vi "Temperature.vi"(0 "physical channels":tag="PXI1Slot2/ai2", 1 "current excitation value":dbl=0.0009 format="%0.5f", 2 "r0":dbl=100.0 format="%0.2f", 5 "current excitation source":i32(ring)=10200 items=["Internal"=10200, "External"=10167, "None"=10230], 7 "resistance configuration":i32(ring)=2 items=["2-Wire"=2, "3-Wire"=3, "4-Wire"=4], 9 "rtd type":i32(ring)=10071 items=["Pt3750"=12481, "Pt3851"=10071, "Pt3911"=12482, "Pt3916"=10069, "Pt3920"=10053, "Pt3928"=12483, "Custom"=10137], 11 "units":i32(ring)=10143 items=["Deg C"=10143, "Deg F"=10144, "Kelvins"=10325, "Deg R"=10145, "From Custom Scale"=10065], 12 "minimum value":dbl format="%0.2f", 13 "maximum value":dbl=100.0 format="%0.2f") -> (4 "data":dbl[](array[numeric]) format="%0.2f", 15 "error out":errorcluster)   [LabVIEW 2019]
uses:
  <vilib>/DAQmx/read.llb/DAQmx Read (Analog 1D DBL NChan 1Samp).vi
  <vilib>/DAQmx/create/channels.llb/DAQmx Create Channel (AI-Temperature-RTD).vi
  <vilib>/DAQmx/miscellaneous.llb/DAQmx Fill In Error Info.vi
panel:
  out "Waveform Chart":dbl[](graph)
  # "Para el NI PXIe-4357"
  # "chanel 2 (ai2) for rtd"
  # "Pt3851 for rtd"
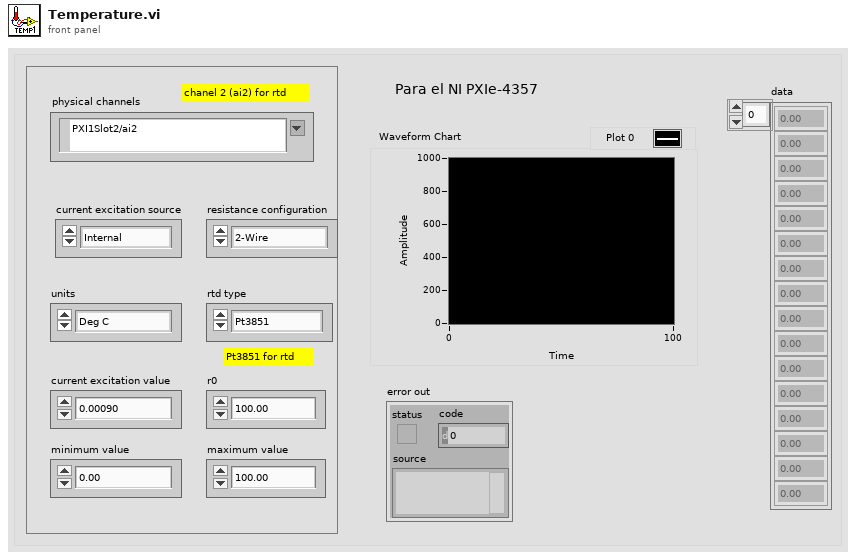
[diagram p1: front panel]
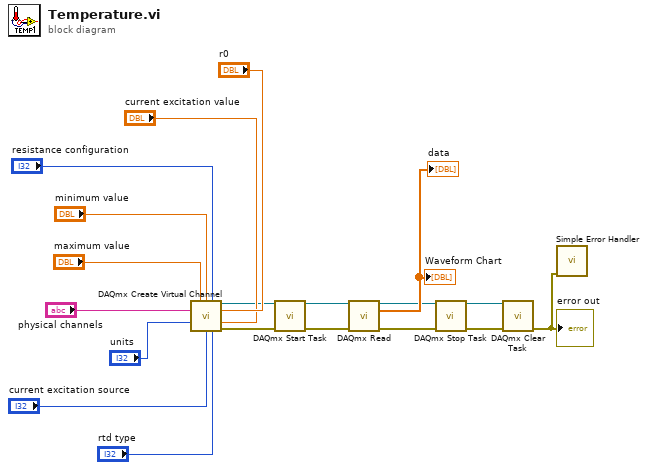
[diagram p0: block diagram]
diagram:
  n1 = call-poly <vilib>:"DAQmx Create Virtual Channel.vi"("maximum value"="maximum value", "minimum value"="minimum value", "resistance configuration"="resistance configuration", "physical channels"="physical channels", "r0"="r0", "units"="units", "current excitation value"="current excitation value", "current excitation source"="current excitation source", "rtd type"="rtd type") -> ("task out"=w3:refnum<k21>, "error out"=w4:errorcluster)  [unwired: 5 in]
  n2 = call <vilib>:"DAQmx Start Task.vi"("task/channels in"=w3, "error in"=w4) -> ("task out"=w5:refnum<k21>, "error out"=w6:errorcluster)  [unwired: 12 in]
  n3 = call-poly <vilib>:"DAQmx Read.vi"("task/channels in"=w5, "error in"=w6) -> ("task out"=w7:refnum<k21>, "data"=→"Waveform Chart" →"data":dbl[], "error out"=w8:errorcluster)  [unwired: 11 in]
  n4 = call <vilib>:"DAQmx Stop Task.vi"("task/channels in"=w7, "error in"=w8) -> ("task out"=w2:refnum<k21>, "error out"=w1:errorcluster)  [unwired: 12 in]
  n5 = call <vilib>:"DAQmx Clear Task.vi"("task in"=w2, "error in"=w1) -> ("error out"=w19:errorcluster)  [unwired: 13 in]
  "error out" <- w19
  n6 = call <vilib>:"Simple Error Handler.vi"("error in (no error)"=w19) -> ()  [unwired: 4 in, 5 out]
